vi "AT Set String A.vi"(8 "error in (no error)":errorcluster, 9 "String":string, 10 "Feature":string, 11 "Handle":i32) -> (0 "error out":errorcluster, 3 "Status":i32)   [LabVIEW 2009]
doc: "Set String\n\nOutput:\n I32 Status\n\nInput:\n I32 Handle\n String Feature\n String Value\n\nThis function will set the value of the specified string feature. The string should be null terminated. An error will be returned if the feature is read only, currently not writable, not a string feature or is not implemented by the camera."
uses:
  atcoreA.dll
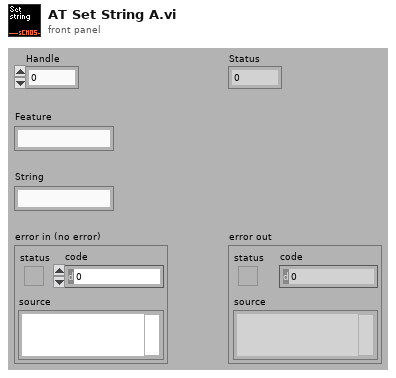
[diagram p1: front panel]
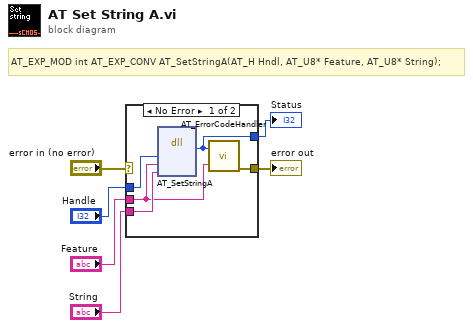
[diagram p0: block diagram]
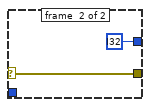
[diagram p2: hidden frame]
diagram:
  # "AT_EXP_MOD int AT_EXP_CONV AT_SetStringA(AT_H Hndl, AT_U8* Feature, AT_U8* String);"
  n1 = case shown="No Error" "error in (no error)" {
    selector: "error in (no error)" -> [_ w13]
    tunnel: [w8 i32 ? ("return type")] -> w6
    tunnel: "Handle" -> [w11 _]
    tunnel: "Feature" -> [w7 _]
    tunnel: "String" -> [w10 _]
    tunnel: [w9 w13] -> w1
    frame #0 {
      n2 = dll-call lib="atcoreA.dll" fn="AT_SetStringA"("Handle"=w11, "Feature"=w7, "String"=w10) -> ("Status"=w8:i32)  [unwired: 6 in, 2 out]
      n3 = call "AT_ErrorCodeHandler.vi"("Error"=w8, "Feature Name"=w7) -> ("error out"=w9:errorcluster)  [unwired: 5 in]
    }
    frame #1 {
    }
  }
  "Status" <- w6
  "error out" <- w1
